vi "Detect unsuported Brick and fall.vi"(10 "Grid":i32[][][](array[numeric]), 11 "Brick Map":map{i32, T1[]}(c390)) -> (1 "Continue":bool, 2 "Grid out":i32[][][](array[numeric]), 3 "Brick Map":map{i32, T1[]}(c390))   [LabVIEW 2023]
uses:
  Cluster_Node.ctl
panel:
  out "left":i32
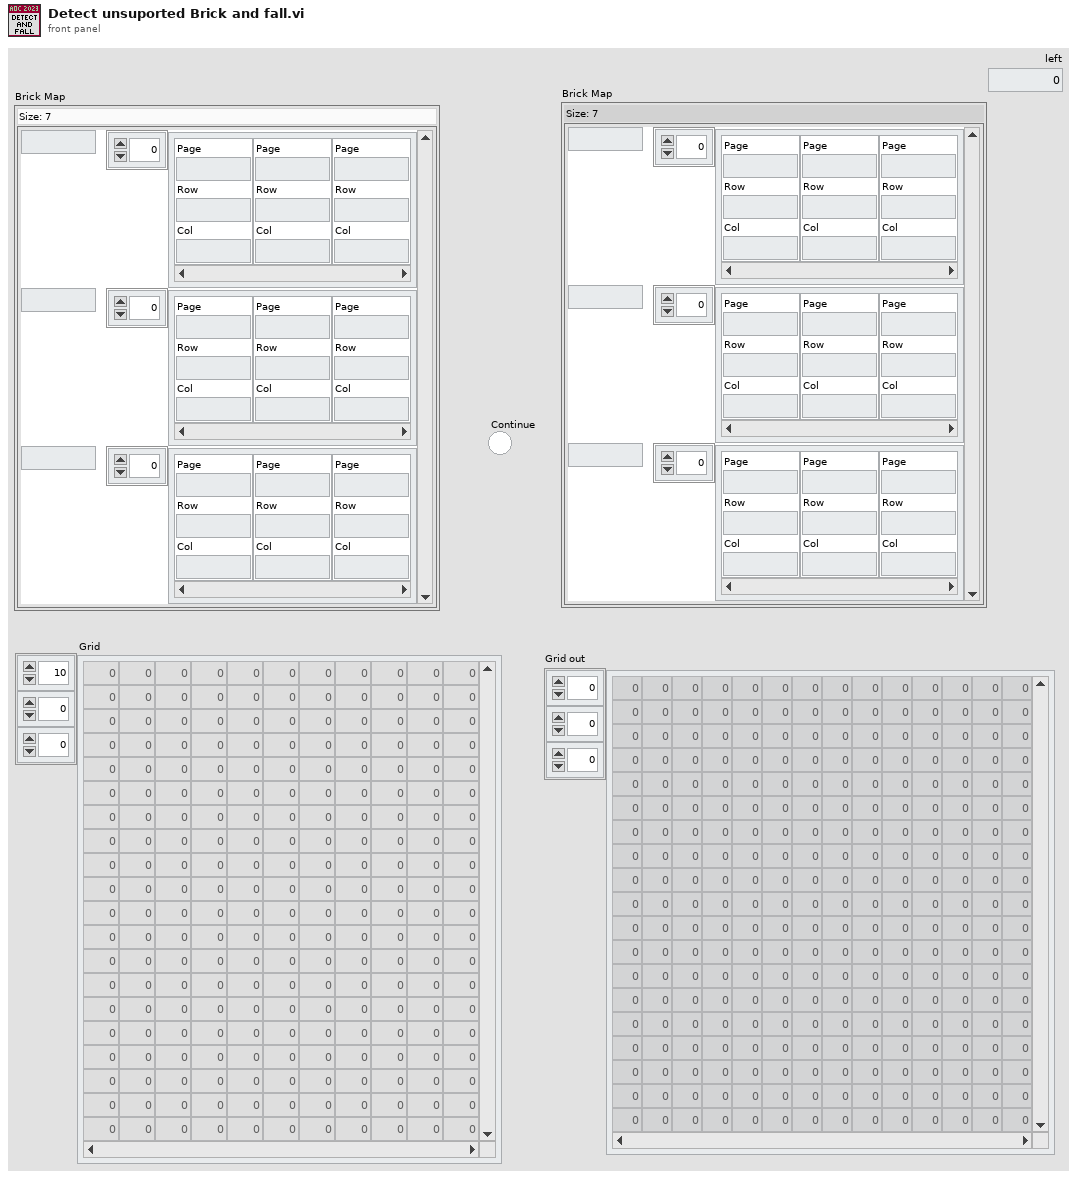
[diagram p1: front panel]
types:
  T1 = typedef "Cluster_Node.ctl" = cluster{"Page":i32, "Row":i32, "Col":i32}
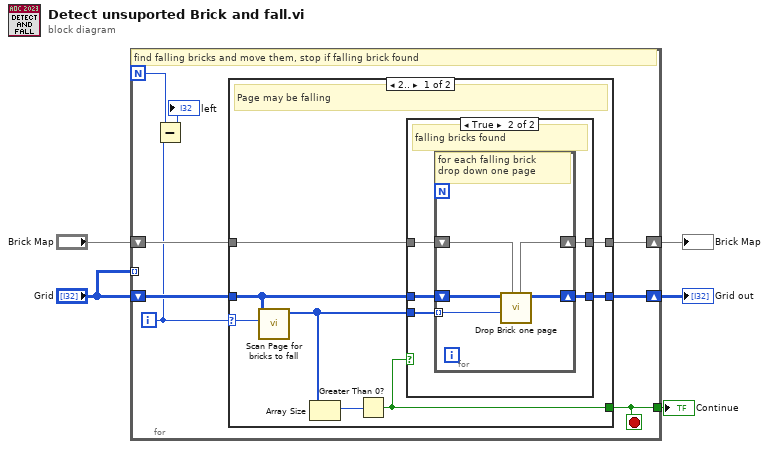
[diagram p0: block diagram]
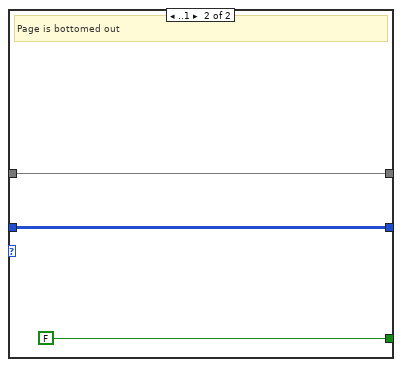
[diagram p3: hidden frame]
diagram:
  n1 = for {
    N -> [w8]
    shift-right: [w10] -> w3
    shift-left: "Grid" -> [w11]
    shift-right: [w12] -> w2
    shift-left: "Brick Map" -> [w13]
    tunnel: [w9] -> w4
    tunnel: "Grid" -> [_] mode=indexing
    i -> [w7]
    stop <- w9 stop-if-true
    # "find falling bricks and move them, stop if falling brick found"
    n2 = Subtract(x=w8, y=w7) -> (x-y=→"left":i32)
    n3 = case shown="2.." w7 {
      selector: w7 -> [w21 _]
      tunnel: [w19 FALSE] -> w9
      tunnel: w13 -> [w18 w36]
      tunnel: [w16 w36] -> w12
      tunnel: w11 -> [w17 w35]
      tunnel: [w15 w35] -> w10
      frame 2.. {
        # "Page may be falling"
        n4 = call "Scan Page for bricks to fall.vi"("Page Index"=w21, "Block Array"=w17) -> ("Fall IDs"=w14:i32[])  [unwired: 9 in]
        n5 = Array Size(array=w14) -> (size(s)=w20:i32)
        n6 = Greater Than 0?(x=w20) -> (x > 0?=w19:bool)
        n7 = case shown="True" w19 {
          tunnel: w18 -> [w23 w27]
          tunnel: w17 -> [w22 w25]
          tunnel: [w23 w26] -> w16
          tunnel: [w22 w24] -> w15
          tunnel: w14 -> [_ w28]
          frame False {
          }
          frame True {
            # "falling bricks found"
            n8 = for {
              tunnel: w28 -> [w33] mode=indexing
              shift-right: [w31] -> w26
              shift-left: w27 -> [w32]
              shift-right: [w29] -> w24
              shift-left: w25 -> [w30]
              # "for each falling brick\ndrop down one page"
              n9 = call "Drop Brick one page.vi"("Map in"=w32, "ID"=w33, "Array in"=w30) -> ("Array out"=w29:i32[][][], "Map out"=w31:map{i32, T1[]})  [unwired: 7 in]
            }
          }
        }
      }
      frame ..1 {
        # "Page is bottomed out"
      }
    }
  }
  "Continue" <- w4
  "Grid out" <- w3
  "Brick Map" <- w2
